vi "mapconf.vi"(11 "map name":T1(ring)=enum."KAIST") -> (1 "y":cluster{dbl, dbl, "y":dbl, "y":dbl, dbl}, 2 "x":cluster{dbl, dbl, "y":dbl, "y":dbl, dbl}, 3 "new picture":picture)   [LabVIEW 2015]
uses:
  <vilib>/picture/picture.llb/imagedata.ctl
  G_ALL.vi
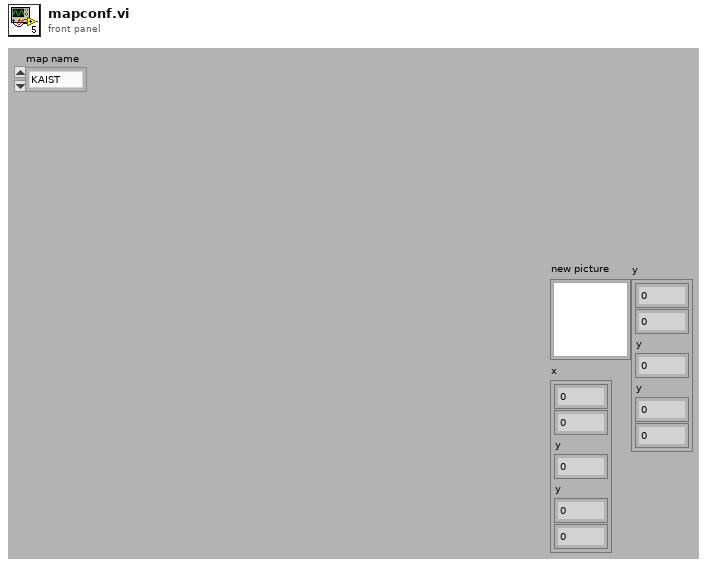
[diagram p1: front panel]
types:
  T1 = enum32{"Namyang", "Hyundai", "KAIST", "Ajou", "Munji", "Airforce", "Car", "KATRI", "Samsung", "Coex", "Gwangnaru", "Inje", "sinjin", "NAVER"}
  T2 = typedef "imagedata.ctl" = cluster{"image type":i32, "image depth":i32, "image":u8[], "mask":u8[], "colors":u32[], "Rectangle":cluster{"left":i16, "top":i16, "right":i16, "bottom":i16}}
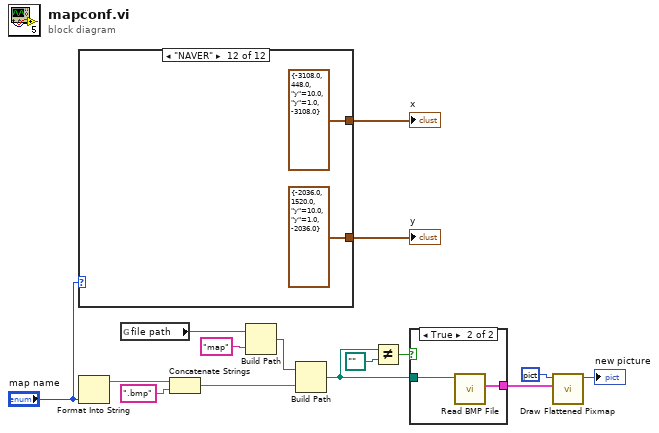
[diagram p0: block diagram]
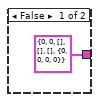
[diagram p2: hidden frame]
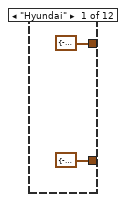
[diagram p3: hidden frame]
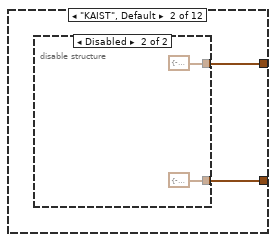
[diagram p4: hidden frame]
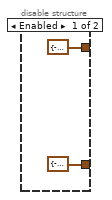
[diagram p5: hidden frame]
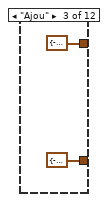
[diagram p6: hidden frame]
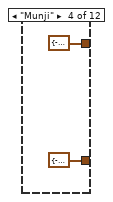
[diagram p7: hidden frame]
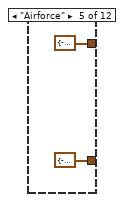
[diagram p8: hidden frame]
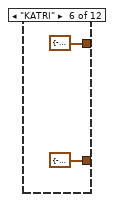
[diagram p9: hidden frame]
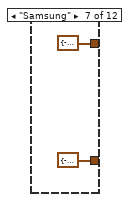
[diagram p10: hidden frame]
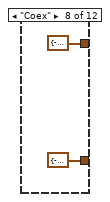
[diagram p11: hidden frame]
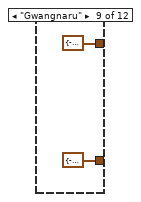
[diagram p12: hidden frame]
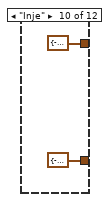
[diagram p13: hidden frame]
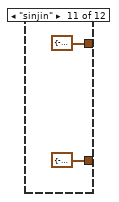
[diagram p14: hidden frame]
diagram:
  n1 = case shown="\"NAVER\"" "map name" {
    tunnel: [cluster{dbl, dbl, "y":dbl, "y":dbl, dbl} {-439.6661, 341.3339, "y"=10.0, "y"=1.0, -439.6661} ("hyundai2_x") w19 cluster{dbl, dbl, "y":dbl, "y":dbl, dbl} {-92.3337125, 135.48694749999999, "y"=10.0, "y"=1.0, -92.3337125} ("ajou_x") cluster{dbl, dbl, "y":dbl, "y":dbl, dbl} {-312.0, 288.0, "y"=10.0, "y"=1.0, -312.0} ("hyundai_x") cluster{dbl, dbl, "y":dbl, "y":dbl, dbl} {-653.415, 142.875, "y"=10.0, "y"=1.0, -653.415} ("hyundai_x") cluster{dbl, dbl, "y":dbl, "y":dbl, dbl} {-818.0, 352.0, "y"=10.0, "y"=1.0, -818.0} ("x") cluster{dbl, dbl, "y":dbl, "y":dbl, dbl} {-81.0, 738.0, "y"=10.0, "y"=1.0, -81.0} ("x") cluster{dbl, dbl, "y":dbl, "y":dbl, dbl} {-2600.0, 1300.0, "y"=10.0, "y"=1.0, -2600.0} ("x") cluster{dbl, dbl, "y":dbl, "y":dbl, dbl} {-101.7435897436, 154.2564102564103, "y"=10.0, "y"=1.0, -101.7435897436} ("x") cluster{dbl, dbl, "y":dbl, "y":dbl, dbl} {-660.0, 640.0, "y"=10.0, "y"=1.0, -660.0} ("x") cluster{dbl, dbl, "y":dbl, "y":dbl, dbl} {-20.5, 138.25, "y"=10.0, "y"=1.0, -20.5} ("Cluster 2") cluster{dbl, dbl, "y":dbl, "y":dbl, dbl} {-3108.0, 448.0, "y"=10.0, "y"=1.0, -3108.0} ("Cluster 2")] -> w15
    tunnel: [cluster{dbl, dbl, "y":dbl, "y":dbl, dbl} {-258.24252, 522.75748, "y"=10.0, "y"=1.0, -258.24252} ("hyundai2_y") w18 cluster{dbl, dbl, "y":dbl, "y":dbl, dbl} {-186.098465, 41.722195, "y"=10.0, "y"=1.0, -186.098465} ("ajou_y") cluster{dbl, dbl, "y":dbl, "y":dbl, dbl} {-189.0, 411.0, "y"=10.0, "y"=1.0, -189.0} ("hyundai_x") cluster{dbl, dbl, "y":dbl, "y":dbl, dbl} {-173.355, 622.935, "y"=10.0, "y"=1.0, -173.355} ("hyundai_x") cluster{dbl, dbl, "y":dbl, "y":dbl, dbl} {-578.0, 592.0, "y"=10.0, "y"=1.0, -578.0} ("Cluster 2") cluster{dbl, dbl, "y":dbl, "y":dbl, dbl} {-323.0, 496.0, "y"=10.0, "y"=1.0, -323.0} ("Cluster 2") cluster{dbl, dbl, "y":dbl, "y":dbl, dbl} {-1983.333, 1916.667, "y"=10.0, "y"=1.0, -1983.333} ("Cluster 2") cluster{dbl, dbl, "y":dbl, "y":dbl, dbl} {-143.3162393162393, 112.6837606837607, "y"=10.0, "y"=1.0, -143.3162393162} ("Cluster 2") cluster{dbl, dbl, "y":dbl, "y":dbl, dbl} {-566.0, 734.0, "y"=10.0, "y"=1.0, -566.0} ("Cluster 2") cluster{dbl, dbl, "y":dbl, "y":dbl, dbl} {-89.25, 69.5, "y"=10.0, "y"=1.0, -89.25} ("Cluster 2") cluster{dbl, dbl, "y":dbl, "y":dbl, dbl} {-2036.0, 1520.0, "y"=10.0, "y"=1.0, -2036.0} ("Cluster 2")] -> w14
    frame "Hyundai" {
    }
    frame "KAIST", Default {
      n2 = disable-structure shown="Disabled" {
        disable-tunnel: [cluster{dbl, dbl, "y":dbl, "y":dbl, dbl} {-523.0, 826.0, "y"=10.0, "y"=1.0, -523.0} ("Cluster") cluster{dbl, dbl, "y":dbl, "y":dbl, dbl} {-19716.6667, 4050.0, "y"=10.0, "y"=1.0, -19716.6667} ("Cluster")] -> w19
        disable-tunnel: [cluster{dbl, dbl, "y":dbl, "y":dbl, dbl} {-1283.0, 66.0, "y"=10.0, "y"=1.0, -1283.0} ("Cluster 2") cluster{dbl, dbl, "y":dbl, "y":dbl, dbl} {-725.0, 13041.6667, "y"=10.0, "y"=1.0, -725.0} ("Cluster 2")] -> w18
        frame Enabled {
        }
        frame Disabled {
        }
      }
    }
    frame "Ajou" {
    }
    frame "Munji" {
    }
    frame "Airforce" {
    }
    frame "KATRI" {
    }
    frame "Samsung" {
    }
    frame "Coex" {
    }
    frame "Gwangnaru" {
    }
    frame "Inje" {
    }
    frame "sinjin" {
    }
    frame "NAVER" {
    }
  }
  "x" <- w15
  "y" <- w14
  n3 = Format Into String("map name") -> (resulting string=w2:string)  [unwired: 3 in, 1 out]
  n4 = global read "G_ALL.vi" "file path"() -> (w5:path)
  n5 = Concatenate Strings(w2, ".bmp") -> (w1:string)
  n6 = Build Path(base path=w5, name or relative path="map") -> (appended path=w7:path)
  n7 = Build Path(base path=w7, name or relative path=w1) -> (appended path=w6:path)
  n8 = Not Equal?(x=w6, y=path "" ("path to BMP file")) -> (x != y?=w11:bool)
  n9 = case shown="True" w11 {
    tunnel: [T2 {"image type"=0, "image depth"=0, "image"=[], "mask"=[], "colors"=[], "Rectangle"={"left"=0, "top"=0, "right"=0, "bottom"=0}} ("image data") w46] -> w10
    tunnel: w6 -> [_ w45]
    frame False {
    }
    frame True {
      n10 = call <vilib>:"Read BMP File.vi"("path to BMP file"=w45) -> ("image data"=w46:T2)  [unwired: 8 in, 2 out]
    }
  }
  n11 = call <vilib>:"Draw Flattened Pixmap.vi"("image data"=w10, "picture"=picture data[5B]) -> ("new picture"=→"new picture":picture)  [unwired: 7 in]
